vi "Read Event Log.vi"(6 "Event Log Path":path, 8 "error in (no error)":errorcluster, 11 "Replay in":refnum<class "Replay.lvclass">) -> (0 "error out":errorcluster, 3 "Replay out":refnum<class "Replay.lvclass">, 4 "Log Data":string[](array[string]))   [LabVIEW 2016, in "CLD Exam - ATM.lvlib" / "Replay.lvclass"]
uses:
  Replay.lvclass
  <vilib>/Utility/file.llb/Read Delimited Spreadsheet (string).vi
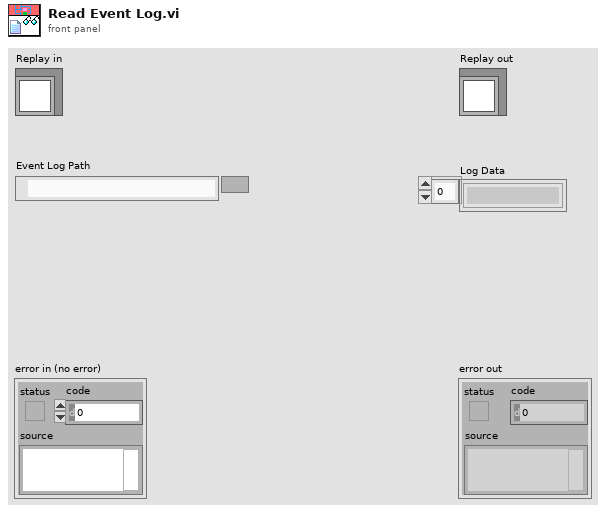
[diagram p1: front panel]
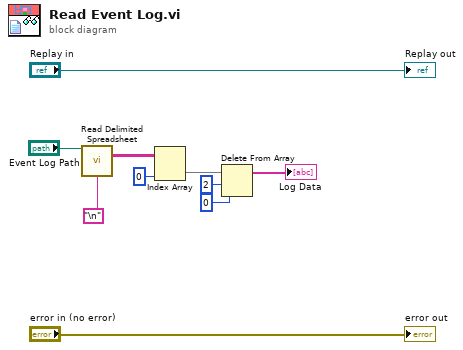
[diagram p0: block diagram]
diagram:
  n1 = call-poly <vilib>:"Read Delimited Spreadsheet.vi"("file path (dialog if empty)"="Event Log Path", "delimiter (\\t)"="\n") -> ("all rows"=w3:string[][])  [unwired: 8 in, 5 out]
  n2 = Index Array(array=w3, index (col)=0 ("disabled index (col)")) -> (element=w2:string[])  [unwired: 1 in]
  n3 = Delete From Array(array=w2, length=2, index=0 ("index (row)")) -> (array with subset deleted=→"Log Data":string[])  [unwired: 1 out]
  "error out" <- "error in (no error)"
  "Replay out" <- "Replay in"
